vi "Report config errors.vi"(6 "SLSC Dynamic Inputs":T1[](array[typedef]), 8 "error in (no error)":errorcluster, 9 "Clear Error?":bool, 11 "Data Value Reference in":refnum<data-value>) -> (0 "error out":errorcluster)   [LabVIEW 2020, in "SLSC EDS Engine.lvlib"]
uses:
  SLSC EDS Engine.lvlib
  SLSC CD API/SLSC CD Engine/SLSC Dynamic Channel.ctl
  SLSC CD API/SLSC CD Engine/SLSC Datatype.ctl
  <vilib>/NI/NIVS Inline Async API/_Data Access Engine/Access Type Classes/Write/Write.lvclass
  <vilib>/NI/NIVS Inline Async API/_Data Access Engine/Access Type Classes/Write/Write.lvclass/Write.ctl
  <vilib>/NI/NIVS Inline Async API/_Data Access Engine/Data Access Engine/Methods/Write.Data.vi
  <vilib>/NI/NIVS Inline Async API/_Data Access Engine/Access Type Classes/Write/Write.ProcessData.vi
  <vilib>/NI/NIVS Inline Async API/_Data Access Engine/Access Type Classes/Write/Write.Buffer.vi
  <vilib>/NI/NIVS Inline Async API/_Data Access Engine/Access Type Classes/Write/Write.Commit.vi
  <vilib>/NI/NIVS Inline Async API/_Data Access Engine/Data Access Engine/Data Access Engine.lvclass
  SLSC CD API/SLSC CD Shared/SLSC CD Shared.lvlib
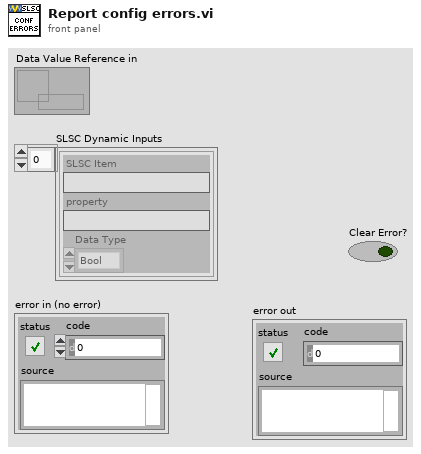
[diagram p1: front panel]
types:
  T1 = typedef "SLSC CD Shared.lvlib/SLSC Dynamic Channel.ctl" = cluster{"SLSC Item":string, "property":string, "Data Type":T2}
  T2 = typedef "SLSC CD Shared.lvlib/SLSC Datatype.ctl" = enum16{"Bool", "Double", "I32", "I64", "String", "U32", "U64"}
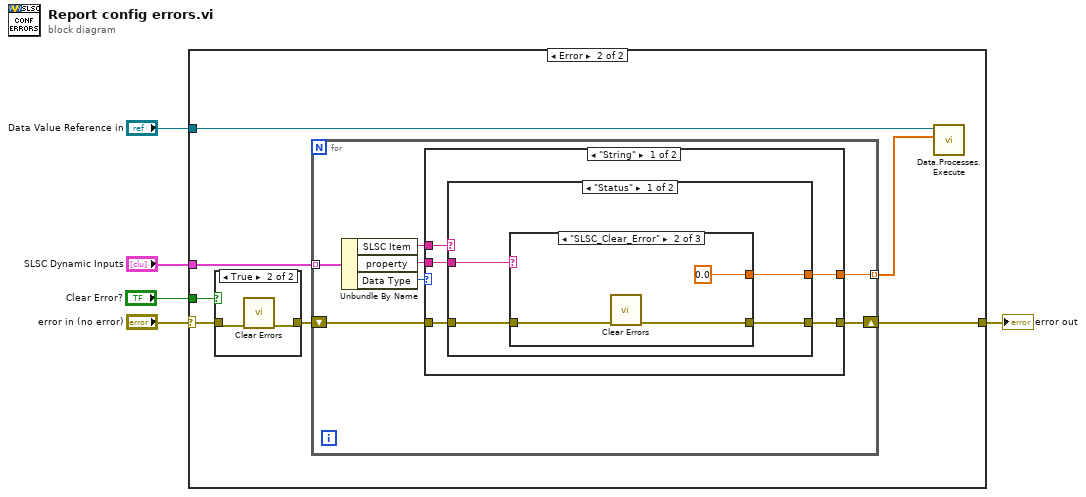
[diagram p0: block diagram]
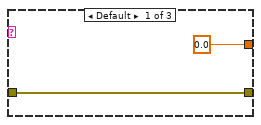
[diagram p4: hidden frame]
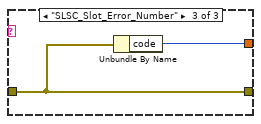
[diagram p5: hidden frame]
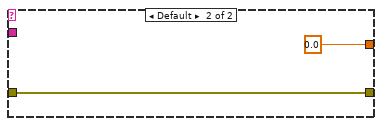
[diagram p6: hidden frame]
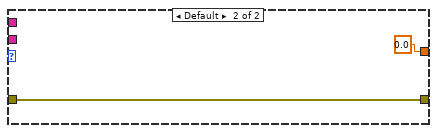
[diagram p7: hidden frame]
diagram:
  n1 = case shown="Error" "error in (no error)" {
    selector: "error in (no error)" -> [w6 w7]
    tunnel: "Data Value Reference in" -> [_ w13]
    tunnel: "SLSC Dynamic Inputs" -> [_ w12]
    tunnel: [w6 w10] -> w2
    tunnel: "Clear Error?" -> [_ w9]
    frame No Error {
    }
    frame Error {
      n2 = case shown="True" w9 {
        tunnel: [w14 w16] -> w8
        tunnel: w7 -> [w14 w15]
        frame False {
        }
        frame True {
          n3 = call <vilib>:"Clear Errors.vi"("error in (no error)"=w15) -> ("error out"=w16:errorcluster)  [unwired: 5 in, 1 out]
        }
      }
      n4 = for {
        tunnel: w12 -> [w23] mode=indexing
        tunnel: [w18] -> w11 mode=indexing
        shift-right: [w17] -> w10
        shift-left: w8 -> [w19]
        n5 = Unbundle By Name(w23) -> ("SLSC Item"=w20:string, "property"=w21:string, "Data Type"=w22:T2)
        n6 = case shown="\"String\"" w22 {
          tunnel: w21 -> [w28 _]
          tunnel: w20 -> [w25 _]
          tunnel: w19 -> [w27 w42]
          tunnel: [w26 0.0 ("LoopDuration(ms)")] -> w18
          tunnel: [w24 w42] -> w17
          frame "String" {
            n7 = case shown="\"Status\"" w25 {
              tunnel: w28 -> [w30 _]
              tunnel: w27 -> [w31 w40]
              tunnel: [w29 w40] -> w24
              tunnel: [w32 0.0 ("LoopDuration(ms)")] -> w26
              frame "Status" {
                n8 = case shown="\"SLSC_Clear_Error\"" w30 {
                  tunnel: [0.0 ("LoopDuration(ms)") 0.0 ("LoopDuration(ms)") w39] -> w32
                  tunnel: w31 -> [w33 w36 w38]
                  tunnel: [w33 w35 w38] -> w29
                  frame Default {
                  }
                  frame "SLSC_Clear_Error" {
                    n9 = call <vilib>:"Clear Errors.vi"("error in (no error)"=w36) -> ("error out"=w35:errorcluster)  [unwired: 5 in, 1 out]
                  }
                  frame "SLSC_Slot_Error_Number" {
                    n10 = Unbundle By Name(w38) -> ("code"=w39:i32)
                  }
                }
              }
              frame Default {
              }
            }
          }
          frame Default {
          }
        }
      }
      n11 = call-poly <vilib>:"Data.Processes.Execute.vi"("Values"=w11, "Ref"=w13) -> ()  [unwired: 9 in, 1 out]
    }
  }
  "error out" <- w2
